vi "kelvinConvert.vi"(1 "Temp hot":dbl) -> (2 "Numeric":dbl)   [LabVIEW 2020]
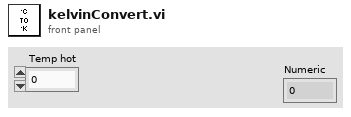
[diagram p1: front panel]
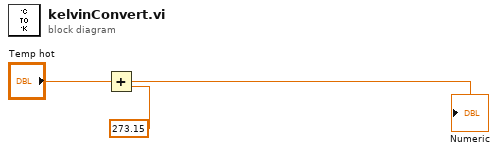
[diagram p0: block diagram]
diagram:
  n1 = Add(x="Temp hot", y=273.15) -> (x+y=→"Numeric":dbl)
